vi "UpdatePaths.vi"(8 "error in (no error)":errorcluster, 11 "Experiment in":refnum<class "Experiment.lvclass">) -> (0 "error out":errorcluster, 3 "Experiment out":refnum<class "Experiment.lvclass">)   [LabVIEW 2014, in "Experiment.lvclass"]
uses:
  Experiment.lvclass
  Experiment.lvclass/Experiment.ctl
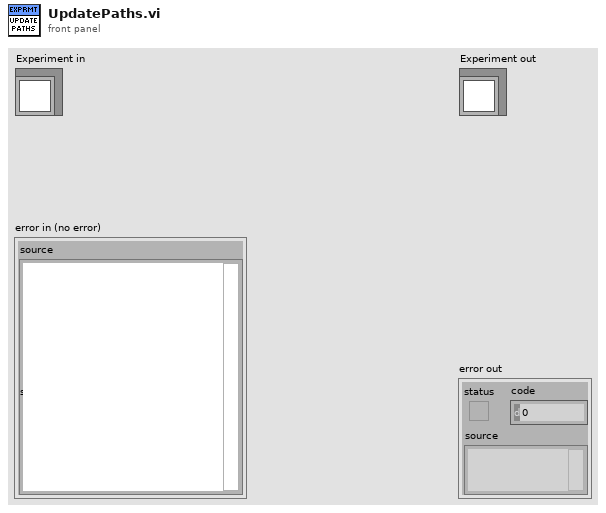
[diagram p1: front panel]
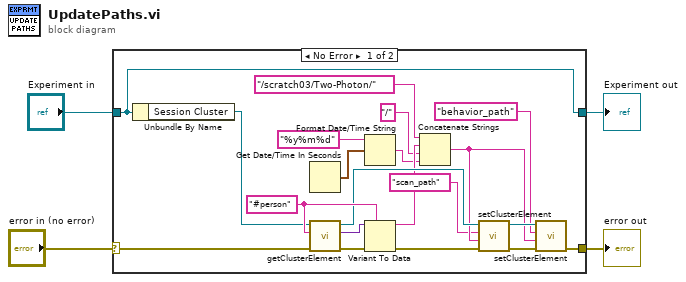
[diagram p0: block diagram]
diagram:
  n1 = case shown="No Error" "error in (no error)" {
    selector: "error in (no error)" -> [w19 w26]
    tunnel: [w20 w26] -> w3
    tunnel: [w5 w25] -> w1
    tunnel: "Experiment in" -> [w5 w25]
    frame No Error {
      w17 = "#person" ("Label.Text")
      n2 = Unbundle By Name(w5) -> ("Session Cluster"=w14:refnum<vi>)
      n3 = Get Date/Time In Seconds() -> (seconds since 1Jan1904=w24:timestamp)
      n4 = call "getClusterElement.vi"("error in (no error)"=w19, "Label.Text"=w17, "reference"=w14) -> ("error out"=w16:errorcluster, "Value"=w18:variant, "reference 2"=w13:refnum<vi>)  [unwired: 6 in]
      n5 = Format Date/Time String(time format string (%c)="%y%m%d", seconds (now)=w24) -> (date/time string=w9:string)  [unwired: 1 out]
      n6 = Variant To Data(error in=w16, type=w17, Variant=w18) -> (data=w11:string, error out=w15:errorcluster)
      n7 = Concatenate Strings("/scratch03/Two-Photon/", w11, "/", w9) -> (w8:string)
      n8 = call "setClusterElement.vi"("error in (no error)"=w15, "Value"=w8, "Label.Text"="scan_path", "reference"=w13) -> ("error out"=w21:errorcluster, "reference 2"=w22:refnum<vi>)  [unwired: 6 in]
      n9 = call "setClusterElement.vi"("error in (no error)"=w21, "Value"=w8, "Label.Text"="behavior_path", "reference"=w22) -> ("error out"=w20:errorcluster)  [unwired: 6 in, 1 out]
    }
    frame Error {
    }
  }
  "error out" <- w3
  "Experiment out" <- w1
